vi "initialise.vi"(8 "error in (no error)":errorcluster) -> (0 "error out":errorcluster, 3 "HardwareList out":refnum<class "HWConfiguration.lvclass">)   [LabVIEW 2009, in "Hardware.lvlib" / "HWControllers.lvlib" / "HWConfiguration.lvclass"]
uses:
  HWConfiguration.lvclass
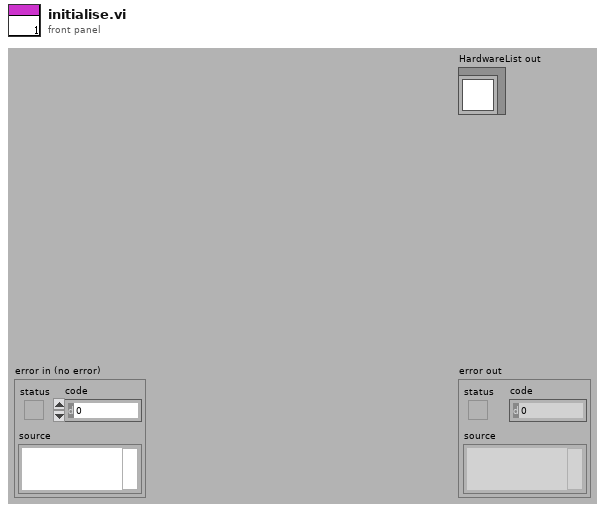
[diagram p1: front panel]
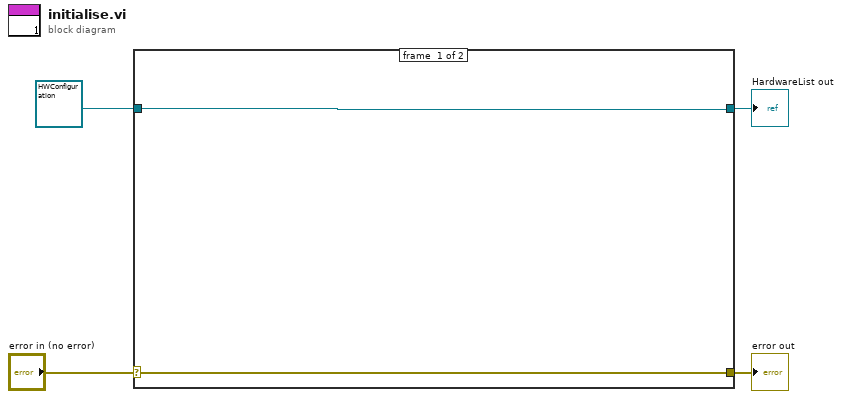
[diagram p0: block diagram]
diagram:
  n1 = case shown="No Error" "error in (no error)" {
    selector: "error in (no error)" -> [w5 w8]
    tunnel: [w5 w8] -> w3
    tunnel: [w6 w7] -> w1
    tunnel: refnum<class "HWConfiguration.lvclass"> refnum ("HardwareList in") -> [w6 w7]
    frame #0 {
    }
    frame #1 {
    }
  }
  "error out" <- w3
  "HardwareList out" <- w1
